vi "Broeadcast Refnum.vi"(8 "error in":errorcluster) -> (0 "error out":errorcluster, 3 "Broadcast Refnum":T1)   [LabVIEW 2020, in "SECS Bridge.lvlib"]
uses:
  SECS Bridge.lvlib
  Broadcast Refnum.ctl
  SECS Communication/HSMS Class/HSMS State.ctl
  <vilib>/Utility/Data Type/NI_Data Type.lvlib
  SECS Communication/HSMS Class/HSMS Class.lvclass
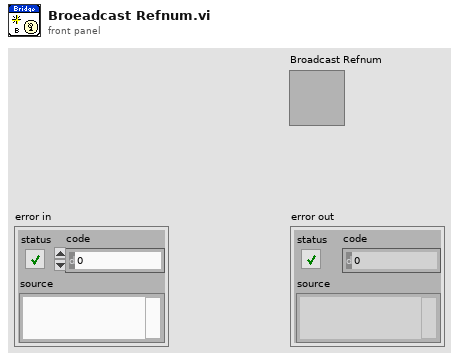
[diagram p1: front panel]
types:
  T1 = typedef "SECS Bridge.lvlib/Broadcast Refnum.ctl" = cluster{"Nottifier Data User Event":refnum<user-event>, "HSMS State User Event":refnum<user-event>, "On-Line User Event":refnum<user-event>}
  T2 = typedef "SECS Communication.lvlib/HSMS Class.lvclass/HSMS State.ctl" = enum16{"[TCP/IP]Not Connect", "[HSMS]Not Selected", "[HSMS]Selected", "Stop"}
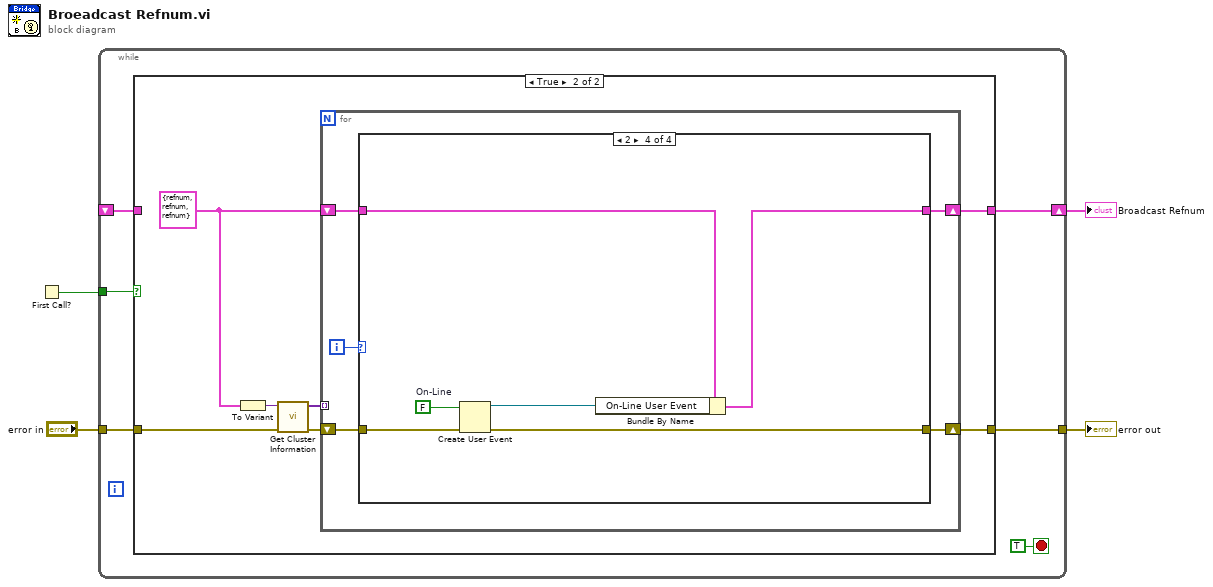
[diagram p0: block diagram]
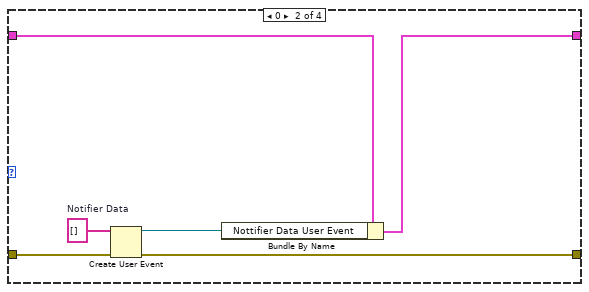
[diagram p4: hidden frame]
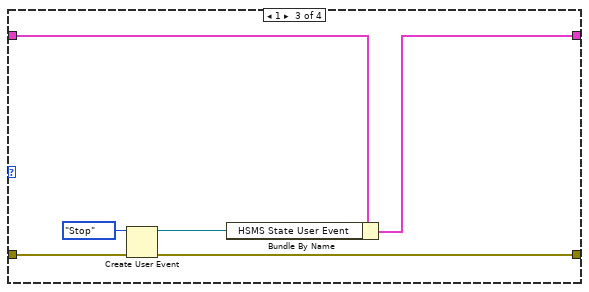
[diagram p5: hidden frame]
diagram:
  n1 = First Call?() -> (First Call?: T/F=w4:bool)
  n2 = while {
    tunnel: "error in" -> [w9]
    tunnel: w4 -> [w10]
    tunnel: [w8] -> w2
    shift-right: [w7] -> w1
    shift-left: _ -> [w6]
    stop <- TRUE stop-if-true
    n3 = case shown="True" w10 {
      tunnel: w9 -> [w11 w19]
      tunnel: [w11 w14] -> w8
      tunnel: [w12 w15] -> w7
      tunnel: w6 -> [w12 _]
      frame False {
      }
      frame True {
        w13 = T1 {"Nottifier Data User Event"=refnum, "HSMS State User Event"=refnum, "On-Line User Event"=refnum} ("Broadcast Refnum")
        n4 = To Variant(anything=w13) -> (Variant=w18:variant)
        n5 = call <vilib>:"Get Cluster Information.vi"("error in (no error)"=w19, "variant"=w18) -> ("error out"=w17:errorcluster, "cluster elements"=w16:variant[])  [unwired: 8 in]
        n6 = for {
          tunnel: w16 -> [_] mode=indexing
          shift-right: [w21] -> w15
          shift-left: w13 -> [w23]
          shift-right: [w20] -> w14
          shift-left: w17 -> [w24]
          i -> [w22]
          n7 = case shown="2" w22 {
            tunnel: w24 -> [w25 w32 w38 w41]
            tunnel: w23 -> [w26 w31 w37 w44]
            tunnel: [w26 w29 w35 w43] -> w21
            tunnel: [w25 w30 w36 w39] -> w20
            frame Default {
            }
            frame 0 {
              w28 = string[] []  # Notifier Data
              n8 = Create User Event(user event datatype=w28, error in=w32) -> (user event=w27:refnum<user-event>, error out=w30:errorcluster)
              n9 = Bundle By Name(cluster=w31, "Nottifier Data User Event"=w27) -> (w29:T1)
            }
            frame 1 {
              n10 = Create User Event(user event datatype=HSMS_State."Stop" ("HSMS State"), error in=w38) -> (user event=w34:refnum<user-event>, error out=w36:errorcluster)
              n11 = Bundle By Name(cluster=w37, "HSMS State User Event"=w34) -> (w35:T1)
            }
            frame 2 {
              w42 = FALSE  # On-Line
              n12 = Create User Event(user event datatype=w42, error in=w41) -> (user event=w40:refnum<user-event>, error out=w39:errorcluster)
              n13 = Bundle By Name(cluster=w44, "On-Line User Event"=w40) -> (w43:T1)
            }
          }
        }
      }
    }
  }
  "Broadcast Refnum" <- w1
  "error out" <- w2
